vi "Response Build.vi"(8 "Content-Type":string, 9 "Content":string, 10 "Headers":map{string, string}(c390), 11 "Status":i32) -> (3 "WSGI Response":T1)   [LabVIEW 2021, in "HttpServer.lvlib"]
uses:
  HttpServer.lvlib
  TypeDefs/WSGI.ctl
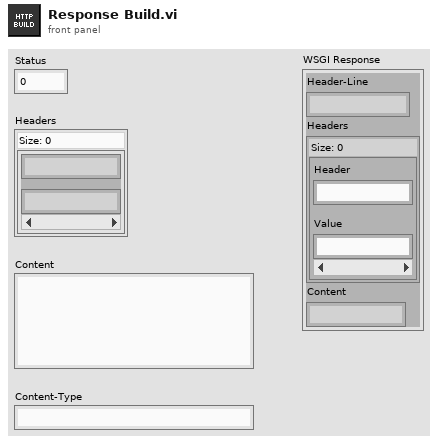
[diagram p1: front panel]
types:
  T1 = typedef "HttpServer.lvlib/WSGI.ctl" = cluster{"Header-Line":string, "Headers":map{string, string}, "Content":string}
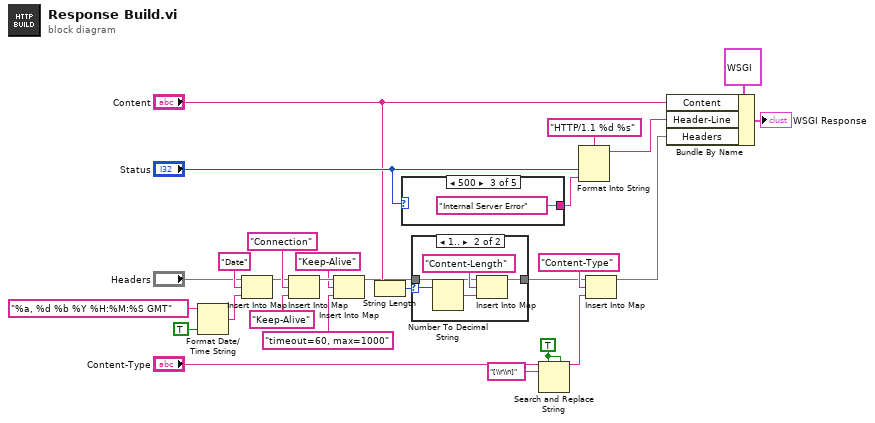
[diagram p0: block diagram]
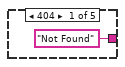
[diagram p2: hidden frame]
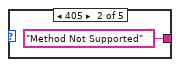
[diagram p3: hidden frame]
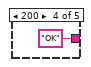
[diagram p4: hidden frame]
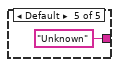
[diagram p5: hidden frame]
diagram:
  w11 = TRUE ("replace all? (F)")
  n1 = Format Date/Time String(time format string (%c)="%a, %d %b %Y %H:%M:%S GMT", UTC format=TRUE) -> (date/time string=w14:string)  [unwired: 1 in]
  n2 = Insert Into Map(map in="Headers", key="Date", value=w14) -> (map out=w2:map{string, string})  [unwired: 2 out]
  n3 = Insert Into Map(map in=w2, key="Connection", value="Keep-Alive") -> (map out=w25:map{string, string})  [unwired: 2 out]
  n4 = Insert Into Map(map in=w25, key="Keep-Alive", value="timeout=60, max=1000") -> (map out=w1:map{string, string})  [unwired: 2 out]
  n5 = String Length(string="Content") -> (length=w18:i32)
  n6 = case shown="500" "Status" {
    tunnel: ["Not Found" "Method Not Supported" "Internal Server Error" "OK" "Unknown"] -> w7
    frame 404 {
    }
    frame 405 {
    }
    frame 500 {
    }
    frame 200 {
    }
    frame Default {
    }
  }
  n7 = case shown="1.." w18 {
    selector: w18 -> [_ w35]
    tunnel: w1 -> [w33 w37]
    tunnel: [w33 w36] -> w19
    frame ..0 {
    }
    frame 1.. {
      n8 = Number To Decimal String(number=w35) -> (decimal integer string=w34:string)  [unwired: 1 in]
      n9 = Insert Into Map(map in=w37, key="Content-Length", value=w34) -> (map out=w36:map{string, string})  [unwired: 2 out]
    }
  }
  n10 = Search and Replace String(replace all?=w11, multiline?=w11, input string="Content-Type", search string="[\\r\\n]") -> (result string=w12:string)  [unwired: 4 in, 3 out]
  n11 = Format Into String(format string="HTTP/1.1 %d %s", "Status", w7) -> (resulting string=w8:string)  [unwired: 2 in, 1 out]
  n12 = Insert Into Map(map in=w19, key="Content-Type", value=w12) -> (map out=w10:map{string, string})  [unwired: 2 out]
  n13 = Bundle By Name(cluster=T1 {"Header-Line"="", "Headers"={}, "Content"=""} ("Http Response"), "Content"="Content", "Header-Line"=w8, "Headers"=w10) -> (→"WSGI Response":T1)
